vi "OAT Timebase Plot (Angle Waveform).vi"(0 "even angle signals":cluster{"r0":dbl, "dr":dbl, "Y":dbl[]}[](array[cluster]) {"r0" format="%.2p"; "dr" format="%.2p"; "Y" format="%.2f"}, 2 "reset? (T)":bool=TRUE, 5 "speed profile":T2 {"speed [RPM]" format="%.2f"; "time [s]" format="%.2f"}, 7 "even angle position info":T3, 9 "revolutions to display [rev]":cluster{"start":dbl, "duration":dbl}={"start"=0.0, "duration"=1.0} {"duration" format="%.2f"; "start" format="%.2f"}, 11 "error in (no error)":errorcluster, 14 "trigger pulse direction":u16(ring)=1 items=["positive going", "negative going"]) -> (4 "X axis":T1, 6 "Y axis":T1, 15 "error out":errorcluster)   [LabVIEW 2017]
uses:
  <vilib>/addons/Sound and Vibration/Order Analysis/Misc/OAT Position Info.ctl
  <vilib>/addons/Sound and Vibration/Order Analysis/Tach Process/SubVIs/speed profile.ctl
  <vilib>/addons/Sound and Vibration/Order Analysis/Backward Compatibility/SubVIs/oa_Timebase Plot Control.ctl
  <vilib>/addons/Sound and Vibration/Order Analysis/Resample Order Tracking/SoundVib_Resampling.lvlib
  <vilib>/addons/Sound and Vibration/Order Analysis/Tach Process/SoundVib_TachProcess.lvlib
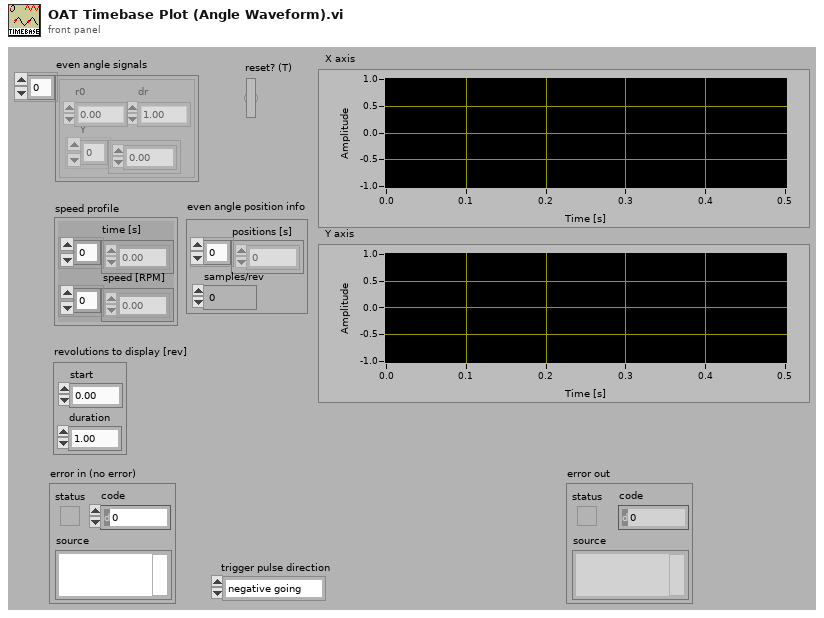
[diagram p1: front panel]
types:
  T1 = typedef "oa_Timebase Plot Control.ctl" = cluster{"X":dbl[], "Y":dbl[]}[]
  T2 = typedef "SoundVib_TachProcess.lvlib/speed profile.ctl" = cluster{"time [s]":dbl[], "speed [RPM]":dbl[]}
  T3 = typedef "OAT Position Info.ctl" = cluster{"positions [s]":dbl[], "samples/rev":dbl}
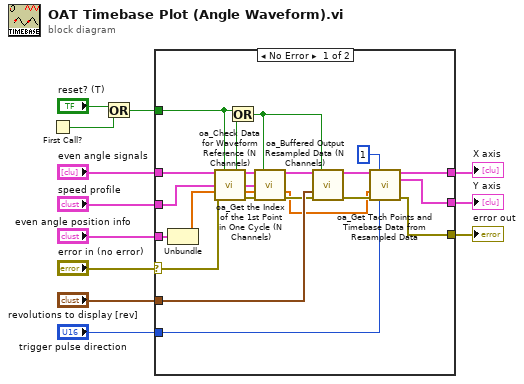
[diagram p0: block diagram]
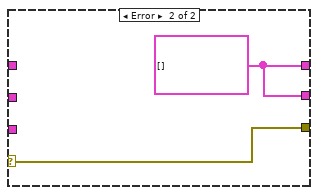
[diagram p2: hidden frame]
diagram:
  n1 = First Call?() -> (First Call?: T/F=w6:bool)
  n2 = Or(x="reset? (T)", y=w6) -> (x .or. y?=w5:bool)
  n3 = case shown="No Error" "error in (no error)" {
    selector: "error in (no error)" -> [w30 w37]
    tunnel: [w19 w37] -> w11
    tunnel: "even angle signals" -> [w31 _]
    tunnel: "speed profile" -> [w29 _]
    tunnel: "even angle position info" -> [w14 _]
    tunnel: w5 -> [w28 _]
    tunnel: "revolutions to display [rev]" -> [w25 _]
    tunnel: "trigger pulse direction" -> [w20 _]
    tunnel: [w17 w36] -> w2
    tunnel: [w16 w36] -> w1
    frame No Error {
      n4 = Unbundle(w14) -> ("positions [s]"=w13:dbl[])  [unwired: 1 out]
      n5 = call <vilib>:"oa_Check Data for Waveform Reference (N Channels).vi"("resampled signal"=w31, "reset? (True)"=w28, "speed profile"=w29, "interpolated pulse positions"=w13, "error in (no error)"=w30) -> ("reset"=w27:bool, "resampled data out"=w34:cluster{"r0":dbl, "dr":dbl, "Y":dbl[]}[], "speed profile out"=w32:T2, "interpolated pulse positions out"=w33:dbl[], "error out"=w35:errorcluster)  [unwired: 3 in, 3 out]
      n6 = Or(x=w28, y=w27) -> (x .or. y?=w23:bool)
      n7 = call <vilib>:"oa_Get the Index of the 1st Point in One Cycle (N Channels).vi"("resampled signal"=w34, "reset? (True)"=w23, "speed profile"=w32, "interpolated pulse positions"=w33, "error in (no error)"=w35) -> ("resampled signal out"=w26:cluster{"r0":dbl, "dr":dbl, "Y":dbl[]}[], "interpolated pulse positions out"=w15:dbl[], "error out"=w24:errorcluster)  [unwired: 8 in]
      n8 = call <vilib>:"oa_Buffered Output Resampled Data (N Channels).vi"("resampled signal in"=w26, "reset? (True)"=w23, "display revolutions"=w25, "error in"=w24) -> ("resampled signal out"=w22:cluster{"r0":dbl, "dr":dbl, "Y":dbl[]}[], "error out"=w21:errorcluster)  [unwired: 9 in, 1 out]
      n9 = call <vilib>:"oa_Get Tach Points and Timebase Data from Resampled Data.vi"("resampled signal in"=w22, "tach duty"=1, "interpolated pulse positions [s]"=w15, "error in"=w21, "trigger pulse direction"=w20) -> ("X axis"=w17:cluster{dbl[], dbl[]}[], "Y axis"=w16:cluster{dbl[], dbl[]}[], "error out"=w19:errorcluster)  [unwired: 8 in]
    }
    frame Error {
      w36 = cluster{dbl[], dbl[]}[] [] ("X axis")
    }
  }
  "error out" <- w11
  "Y axis" <- w1
  "X axis" <- w2
